vi "GOOP400_FindFilesToExchange.vi"(0 "OldClassName(Prefix or suffix for some VIs)":string="NotUsedIfNotWired", 1 "OldFolderPath":path, 2 "NewFolderPath":path, 3 "NewClassName(Prefix or suffix for some VIs)":string="NotUsedIfNotWired") -> (15 "OldFiles":path[](array[path]), 16 "NewFileArray":path[](array[path]))   [LabVIEW 2020]
uses:
  <vilib>/Utility/lvfile.llb/NI_FileType.lvlib
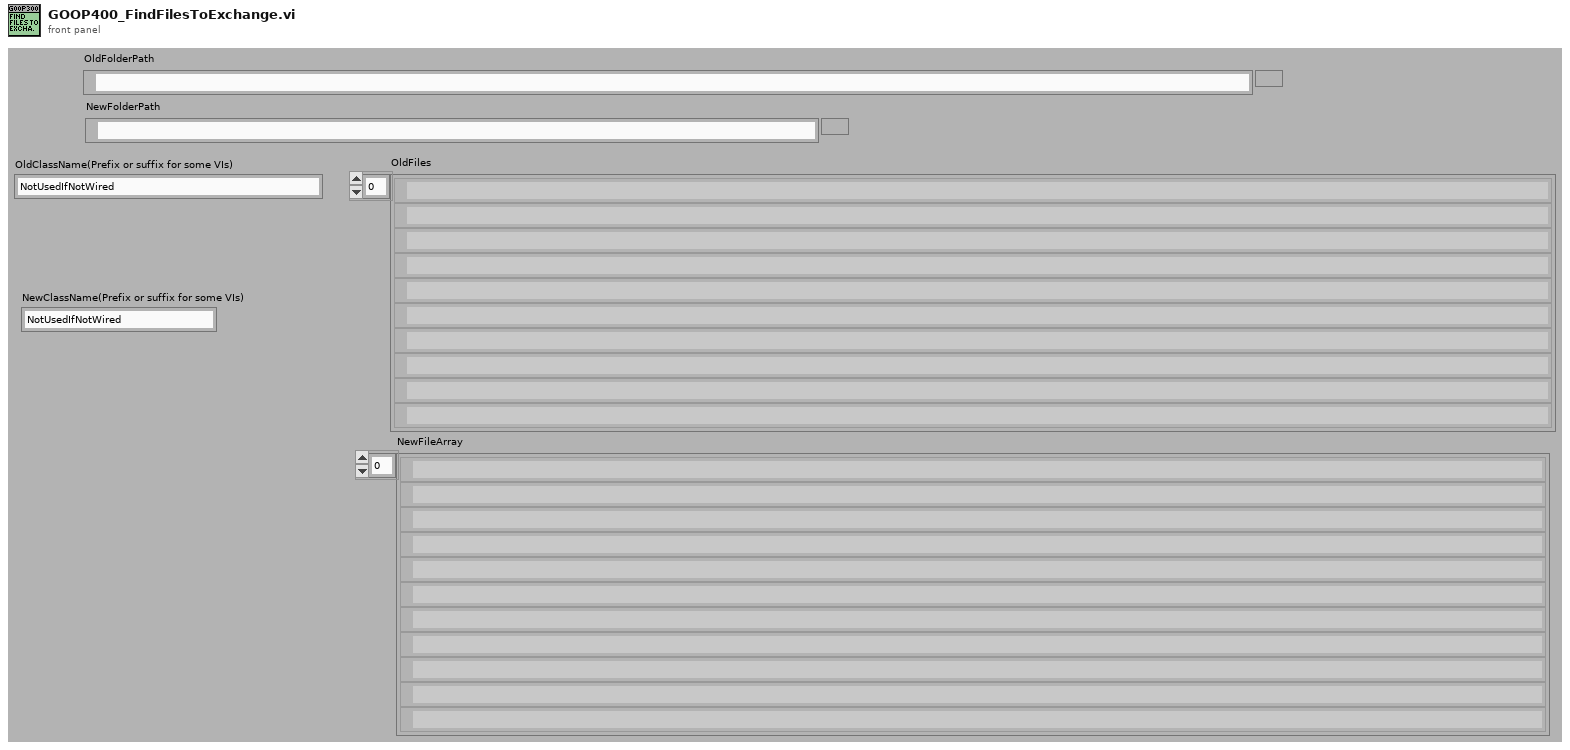
[diagram p1: front panel]
types:
  T1 = typedef "Librarian File List.ctl" = cluster{"name":string, "create date":u32, "mod date":u32, "type":string, "creator":string, "LV version":i32}[]
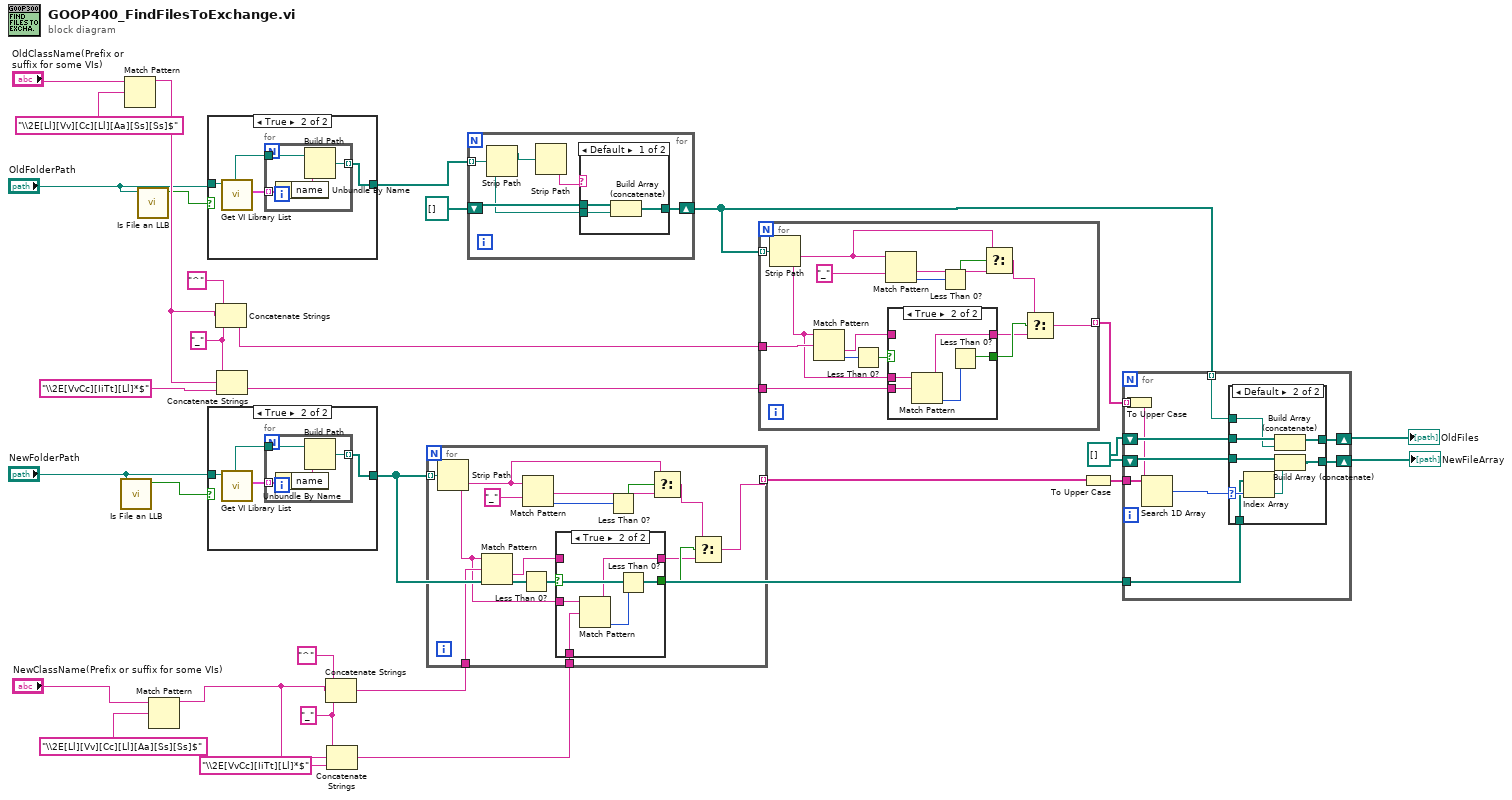
[diagram p0: block diagram]
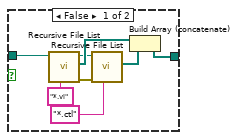
[diagram p2: hidden frame]
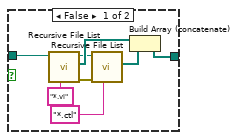
[diagram p3: hidden frame]
diagram:
  w9 = "_" ("regular expression")
  w22 = "_" ("regular expression")
  w26 = path[] []
  n1 = call <vilib>:"Is File an LLB.vi"("path"="NewFolderPath") -> ("Is LLB?"=w4:bool)  [unwired: 9 in, 1 out]
  n2 = Match Pattern(string="OldClassName(Prefix or suffix for some VIs)", regular expression="\\2E[Ll][Vv][Cc][Ll][Aa][Ss][Ss]$") -> (before substring=w8:string)  [unwired: 1 in, 3 out]
  n3 = call <vilib>:"Is File an LLB.vi"("path"="OldFolderPath") -> ("Is LLB?"=w1:bool)  [unwired: 9 in, 1 out]
  n4 = Match Pattern(string="NewClassName(Prefix or suffix for some VIs)", regular expression="\\2E[Ll][Vv][Cc][Ll][Aa][Ss][Ss]$") -> (before substring=w16:string)  [unwired: 1 in, 3 out]
  n5 = case shown="True" w1 {
    tunnel: [w38 w40] -> w3
    tunnel: "OldFolderPath" -> [w31 w39]
    frame False {
      n6 = call <vilib>:"Recursive File List.vi"("pattern"="*.vi", "Folder Path"=w31) -> ("error out"=w35:errorcluster, "All Files in Dir"=w36:path[], "dup Folder Path"=w33:path)  [unwired: 5 in, 2 out]
      n7 = call <vilib>:"Recursive File List.vi"("pattern"="*.ctl", "error in (no error)"=w35, "Folder Path"=w33) -> ("All Files in Dir"=w37:path[])  [unwired: 4 in, 4 out]
      n8 = Build Array (concatenate)(w36, w37) -> (w38:path[])
    }
    frame True {
      n9 = call <vilib>:"Get VI Library List.vi"("library path"=w39) -> ("file list"=w41:T1)  [unwired: 9 in, 1 out]
      n10 = for {
        tunnel: w41 -> [w45] mode=indexing
        tunnel: w39 -> [w43]
        tunnel: [w42] -> w40 mode=indexing
        n11 = Unbundle By Name(w45) -> ("name"=w44:string)
        n12 = Build Path(base path=w43, name or relative path=w44) -> (appended path=w42:path)
      }
    }
  }
  n13 = case shown="True" w4 {
    tunnel: [w53 w55] -> w29
    tunnel: "NewFolderPath" -> [w46 w54]
    frame False {
      n14 = call <vilib>:"Recursive File List.vi"("pattern"="*.vi", "Folder Path"=w46) -> ("error out"=w50:errorcluster, "All Files in Dir"=w51:path[], "dup Folder Path"=w48:path)  [unwired: 5 in, 2 out]
      n15 = call <vilib>:"Recursive File List.vi"("pattern"="*.ctl", "error in (no error)"=w50, "Folder Path"=w48) -> ("All Files in Dir"=w52:path[])  [unwired: 4 in, 4 out]
      n16 = Build Array (concatenate)(w51, w52) -> (w53:path[])
    }
    frame True {
      n17 = call <vilib>:"Get VI Library List.vi"("library path"=w54) -> ("file list"=w56:T1)  [unwired: 9 in, 1 out]
      n18 = for {
        tunnel: w56 -> [w60] mode=indexing
        tunnel: w54 -> [w58]
        tunnel: [w57] -> w55 mode=indexing
        n19 = Unbundle By Name(w60) -> ("name"=w59:string)
        n20 = Build Path(base path=w58, name or relative path=w59) -> (appended path=w57:path)
      }
    }
  }
  n21 = Concatenate Strings("^" ("string"), w8, w9) -> (w7:string)
  n22 = Concatenate Strings(w9, w8, "\\2E[VvCc][IiTt][Ll]*$" ("string")) -> (w6:string)
  n23 = Concatenate Strings("^" ("string"), w16, w22) -> (w23:string)
  n24 = Concatenate Strings(w22, w16, "\\2E[VvCc][IiTt][Ll]*$" ("string")) -> (w19:string)
  n25 = for {
    tunnel: w29 -> [w75] mode=indexing
    tunnel: [w68] -> w30 mode=indexing
    tunnel: w23 -> [w71]
    tunnel: w19 -> [w63]
    n26 = Strip Path(path=w75) -> (name=w61:string)  [unwired: 1 out]
    n27 = Match Pattern(string=w61, regular expression=w71) -> (after substring=w65:string, offset past match=w70:i32)  [unwired: 1 in, 2 out]
    n28 = Less Than 0?(x=w70) -> (x < 0?=w67:bool)
    n29 = Match Pattern(string=w61, regular expression="_") -> (after substring=w62:string, offset past match=w74:i32)  [unwired: 1 in, 2 out]
    n30 = case shown="True" w67 {
      selector: w67 -> [w77 _]
      tunnel: [w77 w82] -> w66
      tunnel: w65 -> [w76 _]
      tunnel: [w76 w81] -> w64
      tunnel: w61 -> [_ w79]
      tunnel: w63 -> [_ w78]
      frame False {
      }
      frame True {
        n31 = Match Pattern(string=w79, regular expression=w78) -> (before substring=w81:string, offset past match=w80:i32)  [unwired: 1 in, 2 out]
        n32 = Less Than 0?(x=w80) -> (x < 0?=w82:bool)
      }
    }
    n33 = Less Than 0?(x=w74) -> (x < 0?=w73:bool)
    n34 = Select(t=w61, s=w73, f=w62) -> (s? t:f=w69:string)
    n35 = Select(t=w69, s=w66, f=w64) -> (s? t:f=w68:string)
  }
  n36 = for {
    tunnel: w3 -> [w83] mode=indexing
    shift-right: [w84] -> w13
    shift-left: path[] [] -> [w85]
    n37 = Strip Path(path=w83) -> (stripped path=w87:path)  [unwired: 1 out]
    n38 = Strip Path(path=w87) -> (name=w86:string)  [unwired: 1 out]
    n39 = case shown="Default" w86 {
      tunnel: w85 -> [w90 w91]
      tunnel: [w89 w91] -> w84
      tunnel: w83 -> [w88 _]
      frame Default {
        n40 = Build Array (concatenate)(w90, w88) -> (w89:path[])
      }
      frame "Methods" {
      }
    }
  }
  n41 = for {
    tunnel: w13 -> [w106] mode=indexing
    tunnel: [w99] -> w12 mode=indexing
    tunnel: w7 -> [w94]
    tunnel: w6 -> [w93]
    n42 = Strip Path(path=w106) -> (name=w92:string)  [unwired: 1 out]
    n43 = Match Pattern(string=w92, regular expression=w94) -> (after substring=w96:string, offset past match=w101:i32)  [unwired: 1 in, 2 out]
    n44 = Less Than 0?(x=w101) -> (x < 0?=w98:bool)
    n45 = Match Pattern(string=w92, regular expression="_") -> (after substring=w104:string, offset past match=w105:i32)  [unwired: 1 in, 2 out]
    n46 = case shown="True" w98 {
      selector: w98 -> [w108 _]
      tunnel: [w108 w113] -> w97
      tunnel: w96 -> [w107 _]
      tunnel: [w107 w112] -> w95
      tunnel: w92 -> [_ w110]
      tunnel: w93 -> [_ w109]
      frame False {
      }
      frame True {
        n47 = Match Pattern(string=w110, regular expression=w109) -> (before substring=w112:string, offset past match=w111:i32)  [unwired: 1 in, 2 out]
        n48 = Less Than 0?(x=w111) -> (x < 0?=w113:bool)
      }
    }
    n49 = Less Than 0?(x=w105) -> (x < 0?=w103:bool)
    n50 = Select(t=w92, s=w103, f=w104) -> (s? t:f=w100:string)
    n51 = Select(t=w100, s=w97, f=w95) -> (s? t:f=w99:string)
  }
  n52 = To Upper Case(1:w30) -> (0:w25:string[])
  n53 = for {
    tunnel: w12 -> [w123] mode=indexing
    tunnel: w25 -> [w116]
    tunnel: w13 -> [w122] mode=indexing
    shift-right: [w120] -> w27
    shift-left: w26 -> [w121]
    shift-right: [w119] -> w28
    shift-left: w26 -> [w118]
    tunnel: w29 -> [w114]
    n54 = To Upper Case(1:w123) -> (0:w117:string)
    n55 = Search 1D Array(1D array=w116, element=w117) -> (index of element=w115:i32)  [unwired: 1 in]
    n56 = case shown="Default" w115 {
      selector: w115 -> [_ w128]
      tunnel: w122 -> [_ w132]
      tunnel: w121 -> [w124 w133]
      tunnel: [w124 w131] -> w120
      tunnel: [w125 w130] -> w119
      tunnel: w118 -> [w125 w129]
      tunnel: w114 -> [_ w127]
      frame -1 {
      }
      frame Default {
        n57 = Index Array(array=w127, index=w128) -> (element=w126:path)
        n58 = Build Array (concatenate)(w133, w132) -> (w131:path[])
        n59 = Build Array (concatenate)(w129, w126) -> (w130:path[])
      }
    }
  }
  "NewFileArray" <- w28
  "OldFiles" <- w27
